vi "Save To File.vi"(8 "error in (no error)":errorcluster, 10 "output settings":T1={"sample rate"=51200.0, "range"=5.0, "terminal configuration"=enum."Pseudodifferential"}, 11 "file path":path) -> (0 "error out":errorcluster)   [LabVIEW 2022 SP3, in "Analog Input Settings.lvlib"]
uses:
  Analog Input Settings.lvlib
  service/generation/controls/analog input settings.ctl
  service/generation/controls/terminal configuration.ctl
  service/generation/controls/AudioGenTypeDefs.lvlib
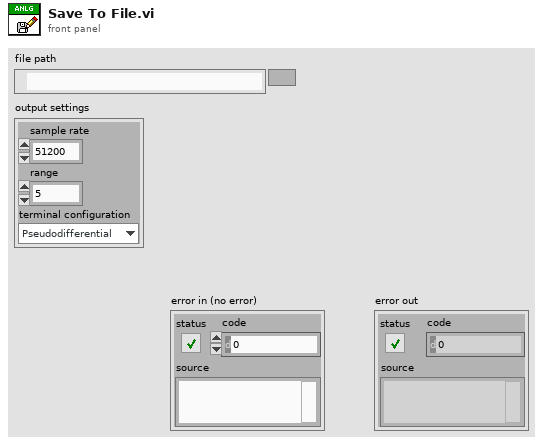
[diagram p1: front panel]
types:
  T1 = typedef "AudioGenTypeDefs.lvlib/analog input settings.ctl" = cluster{"sample rate":dbl, "range":dbl, "terminal configuration":T2}
  T2 = typedef "AudioGenTypeDefs.lvlib/terminal configuration.ctl" = enum32{"Default", "RSE", "Differential", "Pseudodifferential"}
  T3 = typedef "Analog Input Settings.lvlib/analog input settings_json.ctl" = cluster{"sample rate":dbl, "range":dbl, "terminal configuration":string}
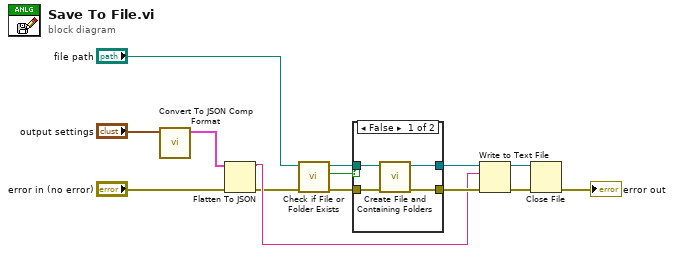
[diagram p0: block diagram]
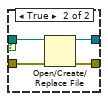
[diagram p2: hidden frame]
diagram:
  n1 = call "Convert To JSON Comp Format.vi"("input settings"="output settings") -> ("input settings JSON"=w2:T3)  [unwired: 10 in]
  n2 = Flatten To JSON(anything=w2, error in (no error)="error in (no error)") -> (JSON string=w8:string, 11:w7:errorcluster)  [unwired: 1 in]
  n3 = call <vilib>:"Check if File or Folder Exists.vi"("error in (no error)"=w7, "path"="file path") -> ("error out"=w5:errorcluster, "file or folder exists?"=w4:bool, "dup path"=w3:path)  [unwired: 7 in]
  n4 = case shown="False" w4 {
    tunnel: [w18 w22] -> w13
    tunnel: [w17 w19] -> w12
    tunnel: w5 -> [w16 w20]
    tunnel: w3 -> [w15 w21]
    frame False {
      n5 = call <vilib>:"Create File and Containing Folders.vi"("error in (no error)"=w16, "file path"=w15) -> ("error out"=w18:errorcluster, "refnum out"=w17:refnum<file>)  [unwired: 8 in]
    }
    frame True {
      n6 = Open/Create/Replace File(file path (use dialog)=w21, error in=w20) -> (refnum out=w19:refnum<file>, error out=w22:errorcluster)  [unwired: 4 in, 1 out]
    }
  }
  n7 = Write to Text File(file (use dialog)=w12, text=w8, error in=w13) -> (refnum out=w10:refnum<file>, error out=w11:errorcluster)  [unwired: 1 in, 1 out]
  n8 = Close File(refnum=w10, error in=w11) -> (error out=→"error out":errorcluster)  [unwired: 1 out]
